vi "CalculateDiscountPercentage.vi"(8 "Error In":errorcluster, 10 "Customer":refnum<class "Customer.lvclass">, 11 "reference in":refnum<class "DiscountCalculator.lvclass">) -> (0 "Error Out":errorcluster, 2 "Return(EXT)":ext, 3 "reference out":refnum<class "DiscountCalculator.lvclass">)   [LabVIEW 2020, in "DiscountCalculator.lvclass"]
uses:
  DiscountCalculator.lvclass
  Customer_class/Customer.lvclass
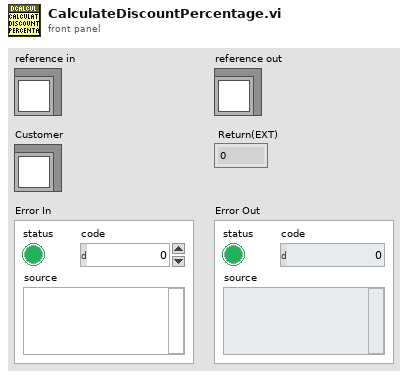
[diagram p1: front panel]
types:
  T1 = typedef "DiscountCalculator.lvclass/ObjectAttributes.ctl" = cluster{"None":bool}
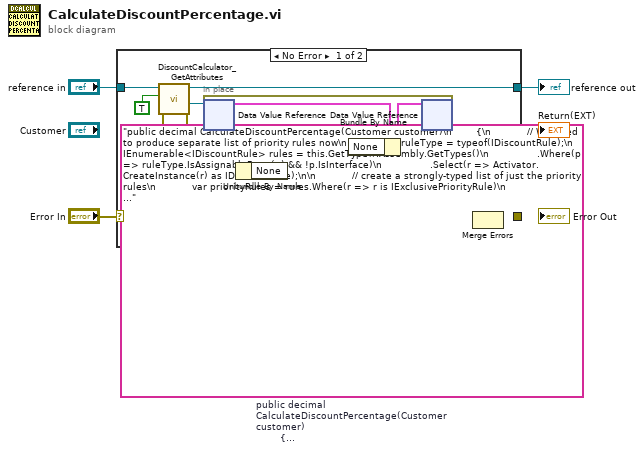
[diagram p0: block diagram]
diagram:
  (unwired) "public decimal CalculateDiscountPercentage(Customer customer)\n        {\n            // We need to produce separate list of priority rules now\n            var ruleType = typeof(IDiscountRule);\n            IEnumerable<IDiscountRule> rules = this.GetType().Assembly.GetTypes()\n                .Where(p => ruleType.IsAssignableFrom(p) && !p.IsInterface)\n                .Select(r => Activator.CreateInstance(r) as IDiscountRule);\n\n            // create a strongly-typed list of just the priority rules\n            var priorityRules = rules.Where(r => r is IExclusivePriorityRule)\n                                     .Select(r => (IExclusivePriorityRule)r)\n                                     .ToList();\n\n            // create a list of all the other rules\n            var baseRules = rules.Where(r => !(r is IExclusivePriorityRule)).ToList();\n\n            var engine = new DiscountRuleEngine(baseRules, priorityRules);\n\n            return engine.CalculateDiscountPercentage(customer);\n        }"  # public decimal CalculateDiscountPercentage(Customer customer)         {             // We need to produce separate list of priority rules now             var ruleType = typeof(IDiscountRule);             IEnumerable<IDiscountRule> rules = this.GetType().Assembly.GetTypes()                 .Where(p => ruleType.IsAssignableFrom(p) && !p.IsInterface)                 .Select(r => Activator.CreateInstance(r) as IDiscountRule);              // create a strongly-typed list of just the priority rules             var priorityRules = rules.Where(r => r is IExclusivePriorityRule)                                      .Select(r => (IExclusivePriorityRule)r)                                      .ToList();              // create a list of all the other rules             var baseRules = rules.Where(r => !(r is IExclusivePriorityRule)).ToList();              var engine = new DiscountRuleEngine(baseRules, priorityRules);              return engine.CalculateDiscountPercentage(customer);         }
  n1 = case shown="No Error" "Error In" {
    selector: "Error In" -> [w11 w16]
    tunnel: [w8 w16] -> w3
    tunnel: [w9 w15] -> w1
    tunnel: "reference in" -> [w12 w15]
    frame No Error {
      n2 = call "DiscountCalculator_GetAttributes.vi"("error in (no error)"=w11, "OnlyGetDvrReference(False)"=TRUE, "reference in"=w12) -> ("error out"=w6:errorcluster, "DataRef"=w7:refnum<data-value>, "reference out"=w9:refnum<class "DiscountCalculator.lvclass">)  [unwired: 5 in, 1 out]
      n3 = in-place {
        n4 = in-place-dvr #1(w7) -> (w13:T1)  [unwired: 1 out]
        n5 = Unbundle By Name(w13) -> ()  [unwired: 1 out]
        n6 = Bundle By Name(cluster=w13) -> (w14:T1)  [unwired: 1 in]
        n7 = in-place-dvr #1(w14) -> (w10:errorcluster)  [unwired: 1 out]
      }
      n8 = Merge Errors(w6, w10) -> (w8:errorcluster)
    }
    frame Error {
    }
  }
  "Error Out" <- w3
  "reference out" <- w1
